vi "例程39-卷积和相关ExpressVI的使用.vi"() -> ()   [LabVIEW 2016]
uses:
  <vilib>/measure/NI_MABase.lvlib
panel:
  in  "停止":bool
  out "波形图X*Y":dynamicdata(graph)=[{"t0"=timestamp(382888.0 s since 1904-01-01), "dt"=0.001, "Y"=array[1999 elements], "attributes"=variant("NI_ChannelName"=variant(string "卷积"))}]
  out "波形图Y":waveform(dbl)(graph)={"t0"=timestamp(382888.0 s since 1904-01-01), "dt"=0.001, "Y"=array[1000 elements]}
  out "波形图X":waveform(dbl)(graph)={"t0"=timestamp(382888.0 s since 1904-01-01), "dt"=0.001, "Y"=array[1000 elements]}
  in  "frequency 2":dbl=10.0 caption="频率" format="%0.2p"
  in  "signal type 2":T1(ring)=enum."Square Wave" caption="信号类型"
  in  "amplitude 2":dbl=8.0 caption="幅值" format="%0.2p"
  in  "phase 2":dbl caption="相位" format="%.2p"
  in  "phase":dbl caption="相位" format="%.2p"
  in  "amplitude":dbl=8.0 caption="幅值" format="%0.2p"
  in  "signal type":T1(ring) caption="信号类型"
  in  "frequency":dbl=10.0 caption="频率" format="%0.2p"
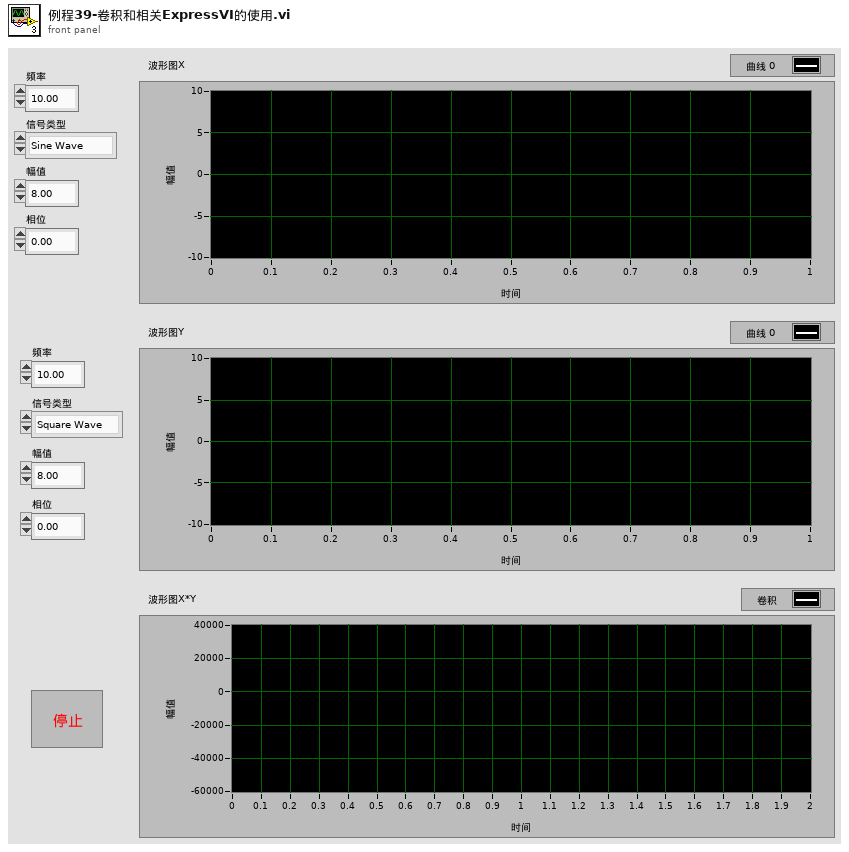
[diagram p1: front panel]
types:
  T1 = enum16{"Sine Wave", "Triangle Wave", "Square Wave", "Sawtooth Wave"}
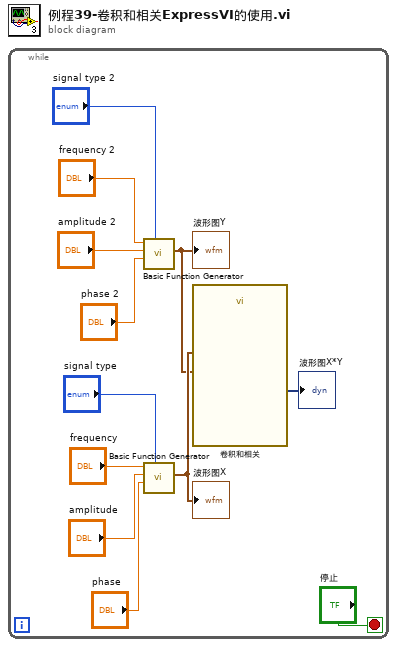
[diagram p0: block diagram]
diagram:
  n1 = while {
    stop <- "停止" stop-if-true
    n2 = call <vilib>:"Basic Function Generator.vi"("signal type"="signal type 2", "phase"="phase 2", "amplitude"="amplitude 2", "frequency"="frequency 2") -> ("signal out"=w2:waveform(dbl))  [unwired: 5 in, 2 out]
    "波形图Y" <- w2
    n3 = call <vilib>:"Basic Function Generator.vi"("signal type"="signal type", "phase"="phase", "amplitude"="amplitude", "frequency"="frequency") -> ("signal out"=w3:waveform(dbl))  [unwired: 5 in, 2 out]
    "波形图X" <- w3
    n4 = call "卷积和相关"("Y"=w2, "X"=w3) -> ("X*Y"=→"波形图X*Y":dynamicdata)  [unwired: 8 in, 1 out]
  }
